vi "Emballage_BDD_verification_test.vi"(8 "Error in":errorcluster caption="Error in (no error)", 9 "ID_ARTICLE":string, 10 "ID_ARTICLE?":bool, 11 "Piece_Scanne":string) -> (0 "Error out":errorcluster, 2 "Chaîne explique_probleme":string, 3 "résultat_valve":bool)   [LabVIEW 2020]
uses:
  Modules/FS/60_FS_Controles/60_FS_SetGet.ctl
panel:
  out "manque test":bool
  out "Tableau Résultat":bool[](array[boolean])
  out "Tableau pas effectué":string[](array[string])
  out "NO_VALVE":string
  out "Result Set":string[][](table) caption="Result Set (from first statement with results)"
  # "IN"
  # "INTERNAL"
  # "OUT"
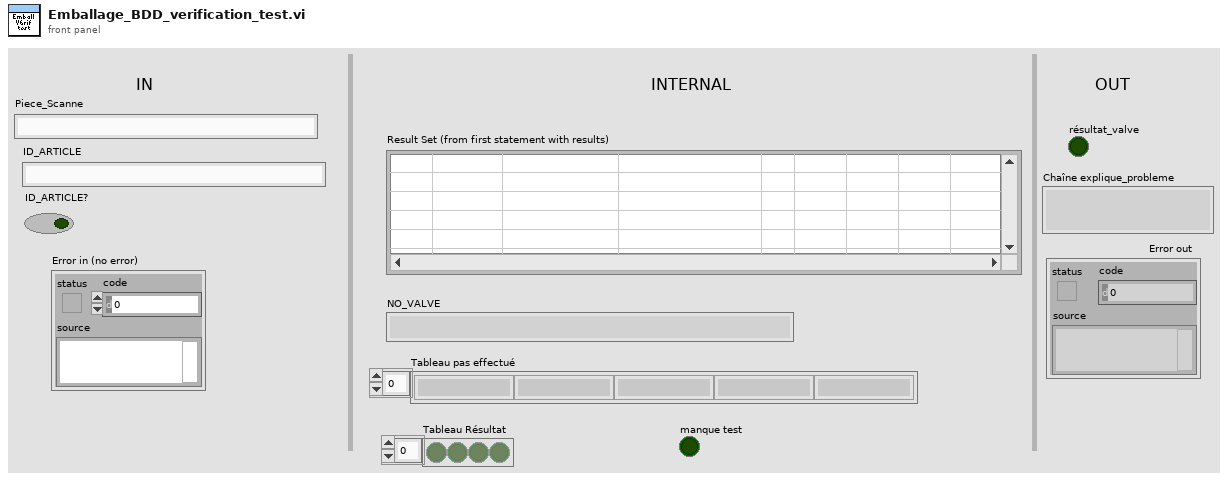
[diagram p1: front panel]
types:
  T1 = typedef "60_FS_SetGet.ctl" = enum16{"set", "get"}
  T2 = typedef "Emballage_BDD_param_Produit.ctl" = cluster{"No_Valve_FAS":string, "suffixe":string, "designation":string, "indice_produit":string, "code_barre_fixe":string, "affiche_code_barre_client":string, "affiche_no_client":string, "Nb_vlve_par_carton":u16, "melange_des_lots_possible":string, "id_article":string, "Indice_Rev":string, "Famille":string, "date":string, "code_barre_fixe_Fin":string, "Longeur_No_Serie":string}
  T3 = typedef "Emballage_Index_correspondance.ctl" = cluster{"Index_CHAMP_RESULTAT":i32, "Index_TABLE_BDD":i32, "Index_CHAMP_ORDRE":i32, "Index_VALEUR_RESULTAT":i32, "Index_FAMILLE_VALVE":i32, "Index_NO_VALVE":i32, "Index_CHAMPS_CONDITION":i32, "Index_VALEUR_CONDITION":i32}
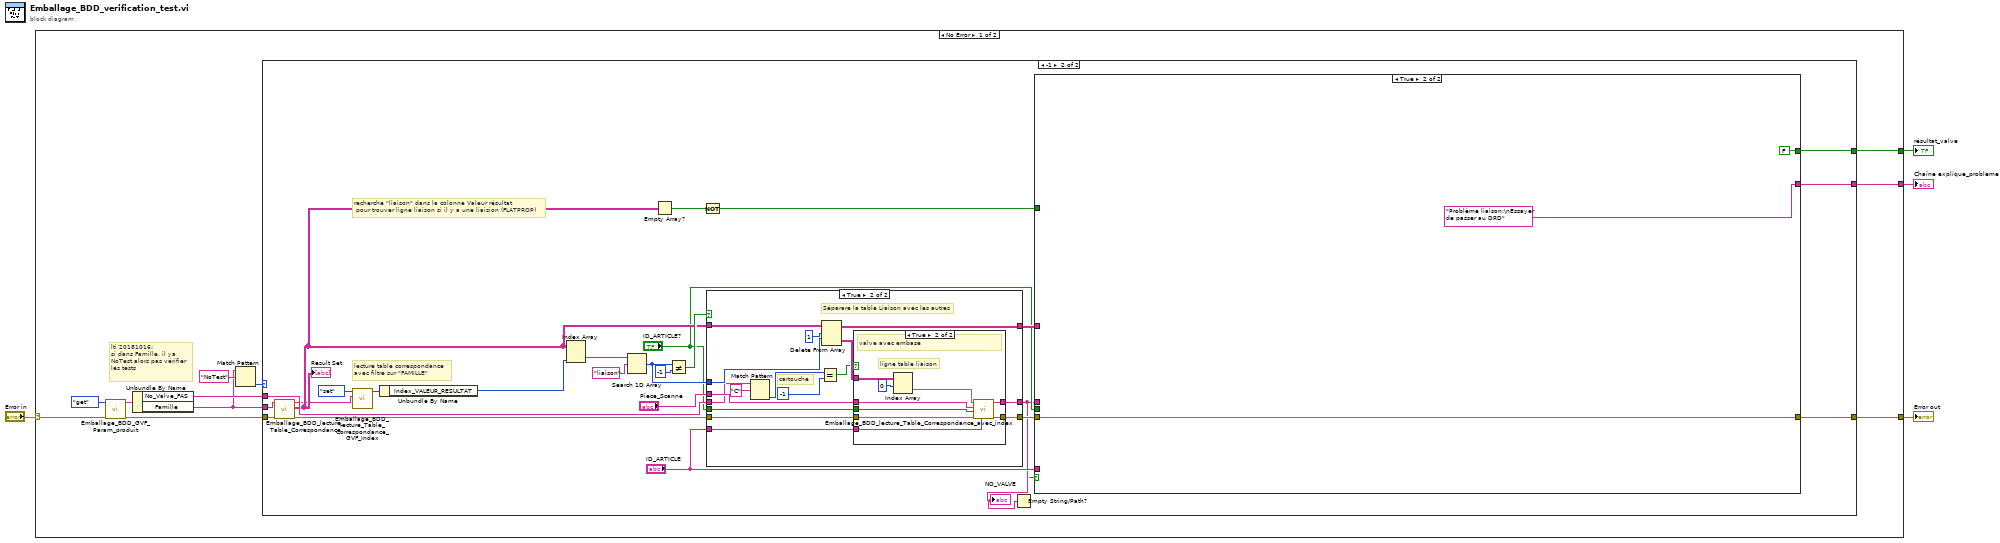
[diagram p0: block diagram]
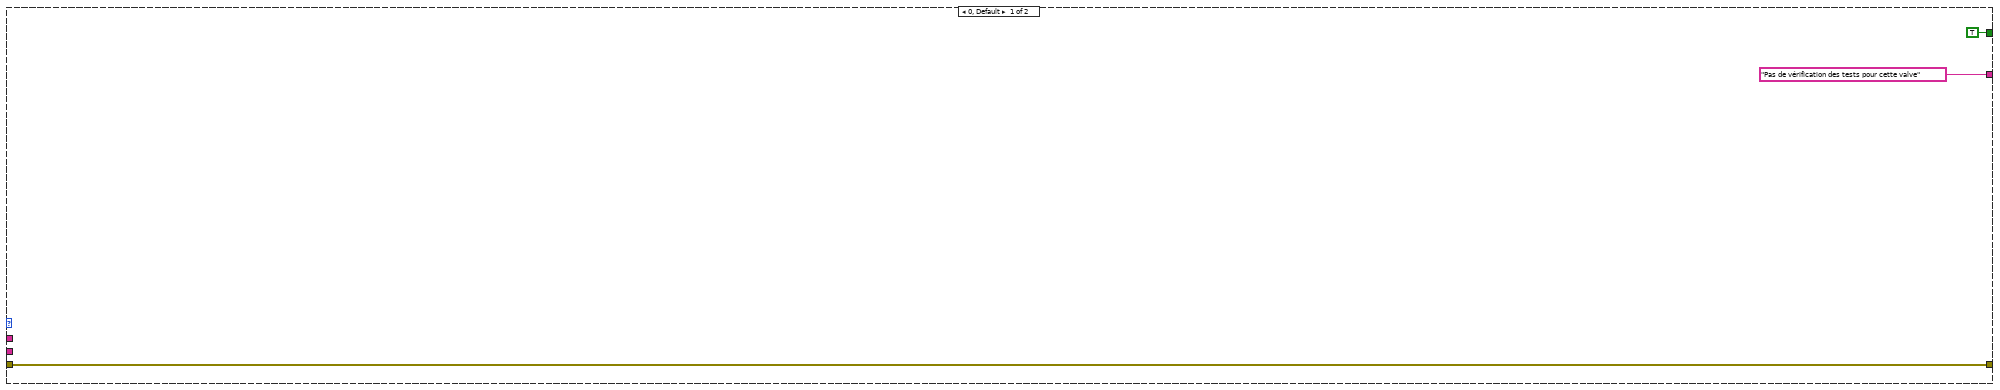
[diagram p2: hidden frame]
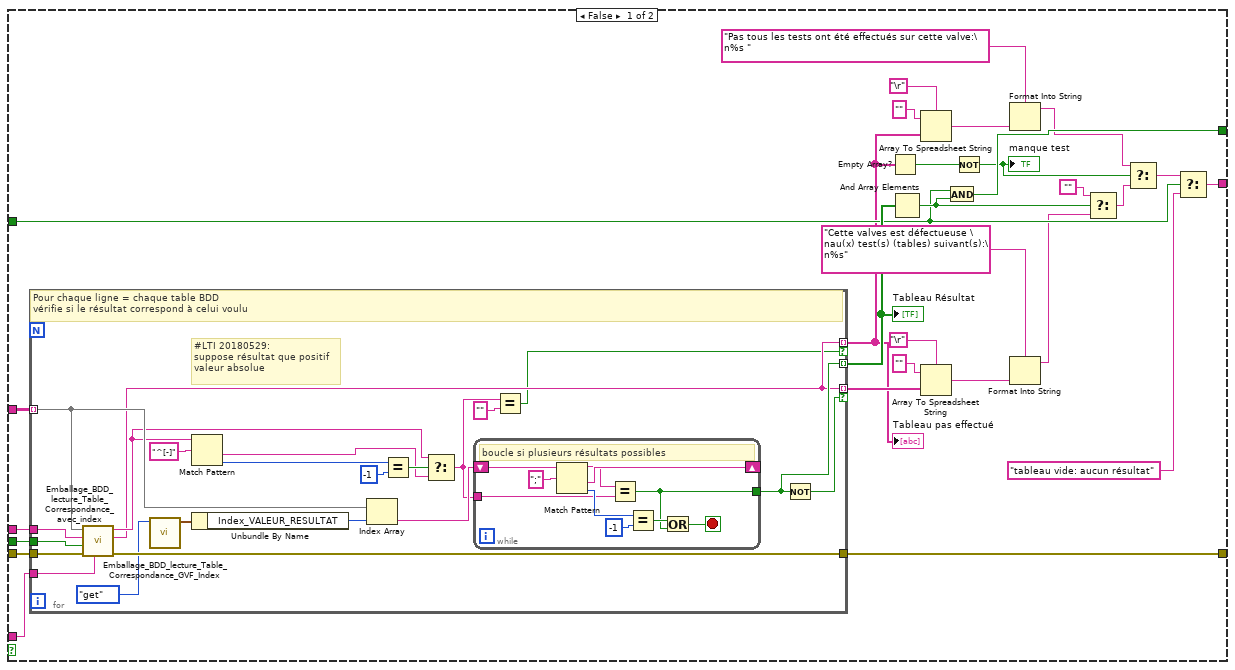
[diagram p3: hidden frame]
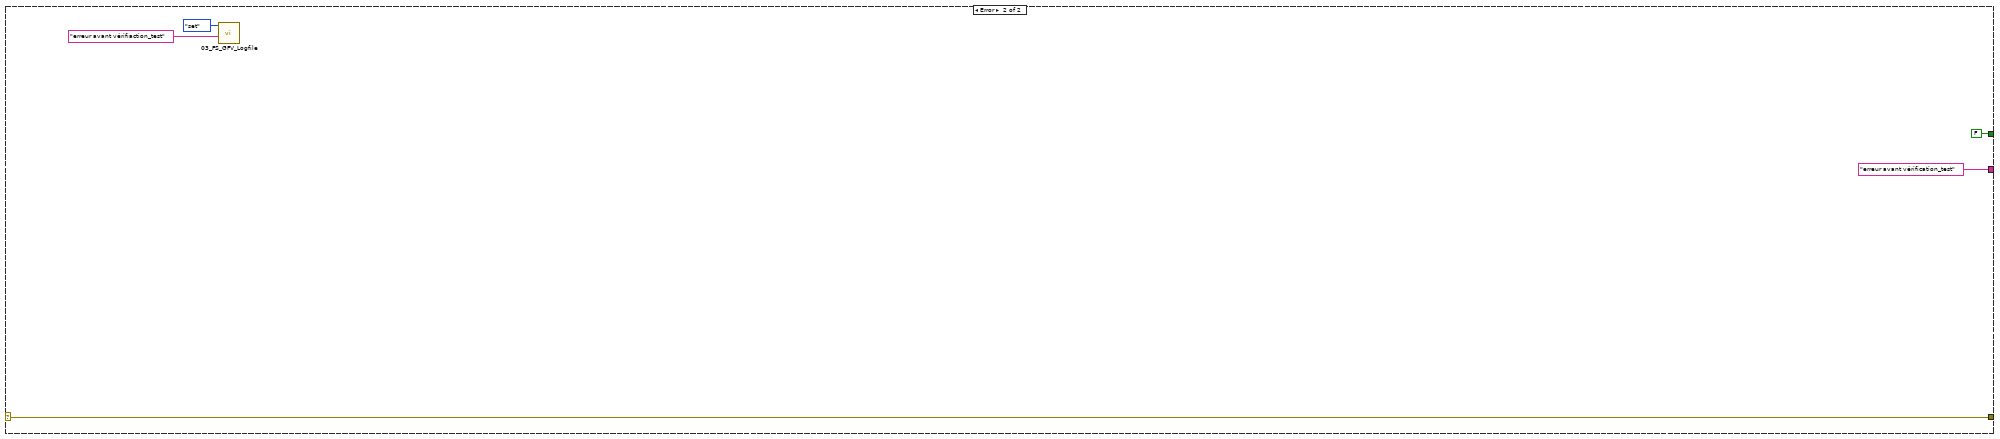
[diagram p6: hidden frame]
diagram:
  n1 = case shown="No Error" "Error in" {
    selector: "Error in" -> [w10 w143]
    tunnel: [w12 w143] -> w4
    tunnel: [w9 "erreur avant vérification_test"] -> w3
    tunnel: [w8 FALSE] -> w1
    frame No Error {
      # "lti 20181016:\nsi dans Famille, il ya \nNoTest alors pas vérifier \nles tests"
      n2 = call "Emballage_BDD_GVF_Param_produit.vi"("Error in"=w10, "Énum"=enum16{"set", "get"}."get") -> ("Error out"=w13:errorcluster, "CLS_param_produit"=w14:T2)  [unwired: 6 in, 2 out]
      n3 = Unbundle By Name(w14) -> ("No_Valve_FAS"=w11:string, "Famille"=w5:string)
      n4 = Match Pattern(string=w5, regular expression="NoTest" ("expression régulière")) -> (offset past match=w6:i32)  [unwired: 1 in, 3 out]
      n5 = case shown="-1" w6 {
        tunnel: w13 -> [w18 w44]
        tunnel: [w18 w43] -> w12
        tunnel: w11 -> [_ w31]
        tunnel: ["Pas de vérification des tests pour cette valve" ("cas faux") w28] -> w9
        tunnel: [TRUE w24] -> w8
        tunnel: w5 -> [_ w23]
        frame 0, Default {
        }
        frame -1 {
          # "lecture table correspondance\navec filtre sur \"FAMILLE\""
          # "recherche \"liaison\" dans la colonne Valeur résultat\n pour trouver ligne liaison si il y a une liaision (FLATPROP)"
          n6 = call "Emballage_BDD_lecture_Table_Correspondance.vi"("entrée d'erreur (pas d'erreur)"=w44, "Famille"=w23) -> ("error out"=w41:errorcluster, "Result Set"=w30:string[][], "Column Names"=w26:string[])  [unwired: 7 in]
          "Result Set" <- w30
          n7 = call "Emballage_BDD_lecture_Table_Correspondance_GVF_Index.vi"("Column Names en entrée"=w26, "Énum"=enum16{"get", "set"}."set") -> ("Cluster_index_champs_correspondance"=w36:T3)  [unwired: 9 in]
          n8 = Unbundle By Name(w36) -> ("Index_VALEUR_RESULTAT"=w38:i32)
          n9 = Index Array(array=w30, index (col)=w38) -> (element=w40:string[])  [unwired: 1 in]
          n10 = Search 1D Array(1D array=w40, element="liaison" ("élément")) -> (index of element=w34:i32)  [unwired: 1 in]
          n11 = Empty Array?(array=w30) -> (empty?=w29:bool)
          n12 = Not Equal?(x=w34, y=-1) -> (x != y?=w32:bool)
          n13 = Not(x=w29) -> (.not. x?=w27:bool)
          n14 = case shown="True" w32 {
            tunnel: w41 -> [w109 w127]
            tunnel: w30 -> [w111 w126]
            tunnel: [w111 w124] -> w37
            tunnel: "Piece_Scanne" -> [w110 w123]
            tunnel: [w110 w122] -> w20
            tunnel: [w109 w121] -> w35
            tunnel: w34 -> [_ w120]
            tunnel: w31 -> [_ w116]
            tunnel: "ID_ARTICLE?" -> [_ w113]
            tunnel: "ID_ARTICLE" -> [_ w112]
            frame False {
            }
            frame True {
              # "cartouche"
              # "Séparare la table Liaison avec les autres"
              n15 = Match Pattern(string=w116, regular expression="C" ("expression régulière")) -> (offset past match=w114:i32)  [unwired: 1 in, 3 out]
              n16 = Equal?(x=w114, y=-1) -> (x = y?=w117:bool)
              n17 = Delete From Array(array=w126, length=1 ("longueur"), index (row)=w120) -> (deleted portion=w125:string[][], array with subset deleted=w124:string[][])  [unwired: 1 in]
              n18 = case shown="True" w117 {
                tunnel: w127 -> [w129 w138]
                tunnel: [w129 w137] -> w121
                tunnel: w123 -> [w128 w135]
                tunnel: [w128 w136] -> w122
                tunnel: w125 -> [_ w133]
                tunnel: w113 -> [_ w131]
                tunnel: w112 -> [_ w130]
                frame False {
                  # "valve cartouche (sans embase)"
                }
                frame True {
                  # "ligne table liaison"
                  # "valve avec embase"
                  n19 = Index Array(array=w133, index (row)=0 ("indice (ligne)")) -> (element=w132:string[])  [unwired: 1 in]
                  n20 = call "Emballage_BDD_lecture_Table_Correspondance_avec_index.vi"("ID_ARTICLE"=w130, "entrée d'erreur (pas d'erreur)"=w138, "ID_ARTICLE?"=w131, "Piece_Scanne"=w135, "ligne_Table_correspondance"=w132) -> ("sortie d'erreur"=w137:errorcluster, "info"=w136:string)  [unwired: 4 in, 1 out]
                }
              }
            }
          }
          "NO_VALVE" <- w20
          n21 = Empty String/Path?(string/path=w20) -> (empty?=w19:bool)
          n22 = case shown="True" w19 {
            tunnel: [w73 w106] -> w43
            tunnel: w37 -> [w68 _]
            tunnel: w20 -> [w66 _]
            tunnel: w35 -> [w65 w106]
            tunnel: [w64 "Problème liaison:\nEssayer de passer au DRD" ("cas faux")] -> w28
            tunnel: w27 -> [w63 _]
            tunnel: [w60 FALSE] -> w24
            tunnel: "ID_ARTICLE?" -> [w54 _]
            tunnel: "ID_ARTICLE" -> [w53 _]
            frame False {
              n23 = for {
                tunnel: w68 -> [w91] mode=indexing
                tunnel: [w75] -> w48 mode=indexing if=w74
                tunnel: [w92] -> w67 mode=indexing
                tunnel: w66 -> [w95]
                tunnel: w65 -> [w94]
                tunnel: [w93] -> w73
                tunnel: [w75] -> w56 mode=indexing if=w90
                tunnel: w54 -> [w79]
                tunnel: w53 -> [w78]
                # "#LTI 20180529:\nsuppose résultat que positif\nvaleur absolue"
                # "Pour chaque ligne = chaque table BDD\nvérifie si le résultat correspond à celui voulu"
                n24 = call "Emballage_BDD_lecture_Table_Correspondance_avec_index.vi"("ID_ARTICLE"=w78, "entrée d'erreur (pas d'erreur)"=w94, "ID_ARTICLE?"=w79, "Piece_Scanne"=w95, "ligne_Table_correspondance"=w91) -> ("sortie d'erreur"=w93:errorcluster, "Table_BDD"=w75:string, "info"=w84:string)  [unwired: 4 in]
                n25 = call "Emballage_BDD_lecture_Table_Correspondance_GVF_Index.vi"("Énum"=enum16{"get", "set"}."get") -> ("Cluster_index_champs_correspondance"=w89:T3)  [unwired: 10 in]
                n26 = Match Pattern(string=w84, regular expression="^[-]" ("chaîne recherchée")) -> (after substring=w83:string, offset past match=w87:i32)  [unwired: 1 in, 2 out]
                n27 = Unbundle By Name(w89) -> ("Index_VALEUR_RESULTAT"=w82:i32)
                n28 = Index Array(array=w91, index=w82) -> (element=w81:string)
                n29 = Equal?(x=w87, y=-1) -> (x = y?=w85:bool)
                n30 = Select(t=w84, s=w85, f=w83) -> (s? t:f=w77:string)
                n31 = while {
                  shift-right: [w100] -> _
                  shift-left: w81 -> [w105]
                  tunnel: w77 -> [w98]
                  tunnel: [w96] -> w92
                  stop <- w97 stop-if-true
                  # "boucle si plusieurs résultats possibles"
                  n32 = Match Pattern(string=w105, regular expression=";" ("expression régulière")) -> (before substring=w99:string, after substring=w100:string, offset past match=w102:i32)  [unwired: 1 in, 1 out]
                  n33 = Equal?(x=w99, y=w98) -> (x = y?=w96:bool)
                  n34 = Equal?(x=w102, y=-1) -> (x = y?=w103:bool)
                  n35 = Or(x=w103, y=w96) -> (x .or. y?=w97:bool)
                }
                n36 = Equal?(x=w77, y="" ("élément")) -> (x = y?=w74:bool)
                n37 = Not(x=w92) -> (.not. x?=w90:bool)
              }
              "Tableau pas effectué" <- w48
              "Tableau Résultat" <- w67
              n38 = Empty Array?(array=w48) -> (empty?=w52:bool)
              n39 = And Array Elements(Boolean array=w67) -> (logical AND=w72:bool)
              n40 = Array To Spreadsheet String(delimiter (Tab)="\r", array=w48, 3:"" ("chaîne de format")) -> (spreadsheet string=w45:string)
              n41 = Array To Spreadsheet String(delimiter (Tab)="\r", array=w56, 3:"" ("chaîne de format")) -> (spreadsheet string=w58:string)
              n42 = And(x=w63, y=w72) -> (x .and. y?=w60:bool)
              n43 = Not(x=w52) -> (.not. x?=w51:bool)
              "manque test" <- w51
              n44 = Format Into String(format string="Pas tous les tests ont été effectués sur cette valve:\n%s ", w45) -> (resulting string=w46:string)  [unwired: 2 in, 1 out]
              n45 = Format Into String(format string="Cette valves est défectueuse \nau(x) test(s) (tables) suivant(s):\n%s", w58) -> (resulting string=w59:string)  [unwired: 2 in, 1 out]
              n46 = Select(t="", s=w72, f=w59) -> (s? t:f=w69:string)
              n47 = Select(t=w46, s=w51, f=w69) -> (s? t:f=w62:string)
              n48 = Select(t=w62, s=w63, f="tableau vide: aucun résultat" ("cas faux")) -> (s? t:f=w64:string)
            }
            frame True {
            }
          }
        }
      }
    }
    frame Error {
      n49 = call "03_FS_GFV_Logfile.vi"("Chaîne"="erreur avant vérifiaction_test", "States"=60_FS_SetGet."set") -> ()  [unwired: 8 in, 2 out]
    }
  }
  "Error out" <- w4
  "Chaîne explique_probleme" <- w3
  "résultat_valve" <- w1
